vi "DB Float Array.vi"() -> (3 "DB Int Array":sgl[](array[numeric]))   [LabVIEW 2017, in "Database.lvlib"]
uses:
  Database.lvlib
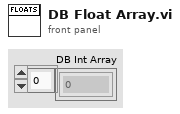
[diagram p1: front panel]
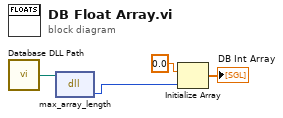
[diagram p0: block diagram]
diagram:
  n1 = call "Database DLL Path.vi"() -> ("DLL Path"=w3:path)  [unwired: 5 in]
  n2 = dll-call lib="?" fn="max_array_length"(path in=w3) -> ("return type"=w2:i32)  [unwired: 2 in, 2 out]
  n3 = Initialize Array(sgl 0.0 ("element"), w2) -> (→"DB Int Array":sgl[])
